vi "EditorThumbnail setRefnum.vi"(8 "error in (no error)":errorcluster, 10 "clusterRefnum":T1, 11 "EditorThumbnail in":refnum<class "EditorThumbnail.lvclass">) -> (0 "error out":errorcluster, 3 "EditorThumbnail out":refnum<class "EditorThumbnail.lvclass">)   [LabVIEW 2018, in "EditorThumbnail.lvclass"]
uses:
  EditorThumbnail.lvclass
  EditorThumbnail.lvclass/EditorThumbnail.ctl
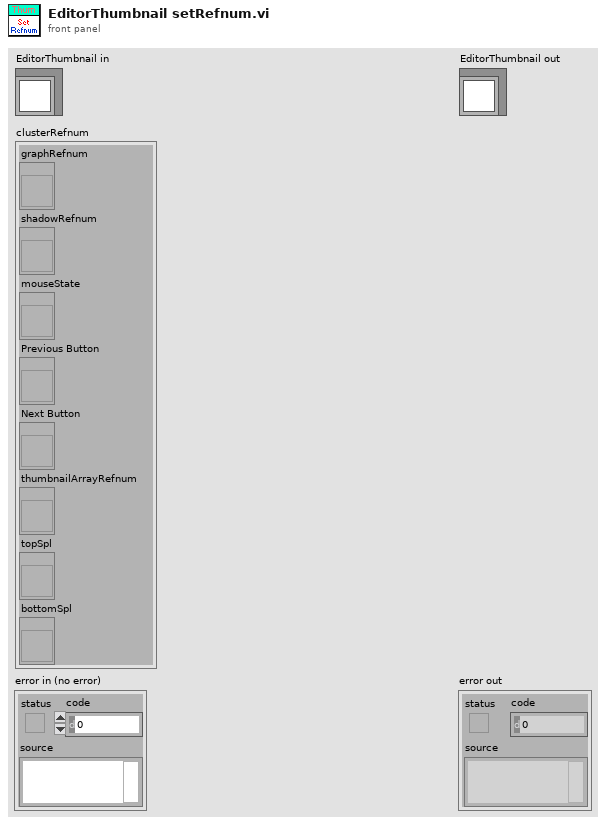
[diagram p1: front panel]
types:
  T1 = cluster{"graphRefnum":refnum<vi>, "shadowRefnum":refnum<vi>, "mouseState":refnum<vi>, "Previous Button":refnum<vi>, "Next Button":refnum<vi>, "thumbnailArrayRefnum":refnum<vi>, "topSpl":refnum<vi>, "bottomSpl":refnum<vi>}
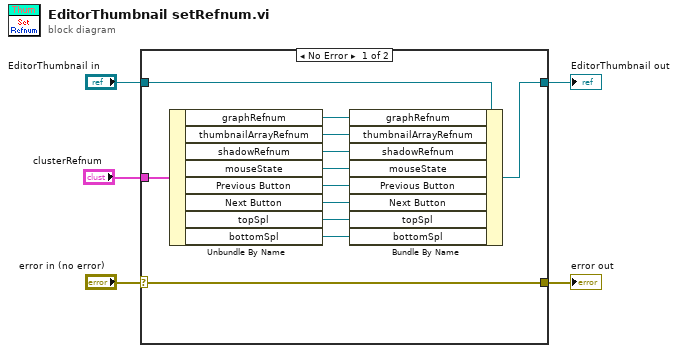
[diagram p0: block diagram]
diagram:
  n1 = case shown="No Error" "error in (no error)" {
    selector: "error in (no error)" -> [w17 w19]
    tunnel: [w17 w19] -> w4
    tunnel: [w15 w18] -> w2
    tunnel: "EditorThumbnail in" -> [w16 w18]
    tunnel: "clusterRefnum" -> [w12 _]
    frame No Error {
      n2 = Unbundle By Name(w12) -> ("graphRefnum"=w14:refnum<vi>, "thumbnailArrayRefnum"=w8:refnum<vi>, "shadowRefnum"=w13:refnum<vi>, "mouseState"=w11:refnum<vi>, "Previous Button"=w10:refnum<vi>, "Next Button"=w9:refnum<vi>, "topSpl"=w7:refnum<vi>, "bottomSpl"=w6:refnum<vi>)
      n3 = Bundle By Name(cluster=w16, "graphRefnum"=w14, "thumbnailArrayRefnum"=w8, "shadowRefnum"=w13, "mouseState"=w11, "Previous Button"=w10, "Next Button"=w9, "topSpl"=w7, "bottomSpl"=w6) -> (w15:refnum<class "EditorThumbnail.lvclass">)
    }
    frame Error {
    }
  }
  "error out" <- w4
  "EditorThumbnail out" <- w2
